vi "DAQNavi Read (Digital 2D U8 NChan NSamp).vi"(8 "error in (no error)":errorcluster, 9 "number of samples per channel to read":u32=1000, 10 "timeout":dbl=10.0 format="%0.2f", 11 "task in":i32) -> (0 "error out":errorcluster, 2 "data":u8[][](array[numeric]), 3 "task out":i32)   [LabVIEW 2020]
uses:
  DAQNavi_LV.dll
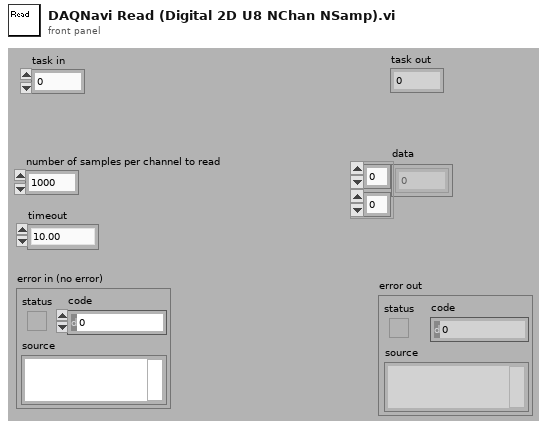
[diagram p1: front panel]
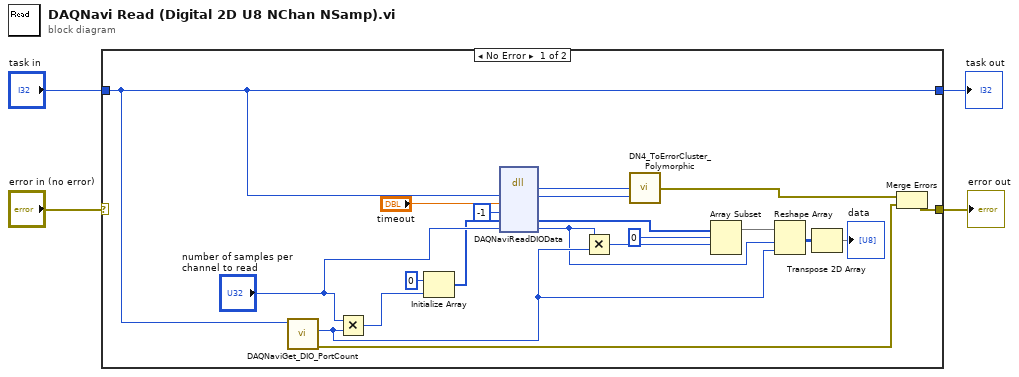
[diagram p0: block diagram]
diagram:
  n1 = case shown="No Error" "error in (no error)" {
    selector: "error in (no error)" -> [_ w25]
    tunnel: "task in" -> [w20 w26]
    tunnel: [w20 w26] -> w2
    tunnel: [w18 w25] -> w1
    frame No Error {
      n2 = call "DAQNaviGet_DIO_PortCount.vi"("task in"=w20) -> ("error out"=w16:errorcluster, "port count"=w11:i32)  [unwired: 1 in, 8 out]
      n3 = Multiply(x="number of samples per channel to read", y=w11) -> (x*y=w19:u32)
      n4 = Initialize Array(u8 0 ("element"), w19) -> (w8:u8[])
      n5 = dll-call lib="DAQNavi_LV.dll" fn="DAQNaviReadDIOData"("taskID"=w20, "timeout"="timeout", "portBit"=-1, "portData"=w8, "samples"="number of samples per channel to read") -> ("return type"=w22:i32, "taskID"=w6:i32, "portData"=w7:u8[], "samples"=w10:u32)  [unwired: 5 in, 2 out]
      n6 = Multiply(x=w10, y=w11) -> (x*y=w12:u32)
      n7 = call "DN4_ToErrorCluster_Polymorphic.vi"("task id"=w6, "error code"=w22) -> ("error out"=w17:errorcluster)  [unwired: 3 out]
      n8 = Array Subset(array=w7, index=0, length=w12) -> (w15:u8[])
      n9 = Reshape Array(w15, w10, w11) -> (w14:u8[][])
      n10 = Transpose 2D Array(2D array=w14) -> (transposed array=→"data":u8[][])
      n11 = Merge Errors(w17, w16) -> (w18:errorcluster)
    }
    frame Error {
    }
  }
  "task out" <- w2
  "error out" <- w1
